vi "niRFUtil LCAPI Copy 1D Array (1 I8).vi"(0 "Source0 1D Array (I8)":i8[](array[numeric]), 11 "error in (no error)":errorcluster, 12 "Data Copy Descriptor":u64) -> (4 "Source0 1D Array (I8) Out":i8[](array[numeric]), 15 "error out":errorcluster)   [LabVIEW 2015, in "niRFUtil.lvlib"]
uses:
  niRFUtil.lvlib
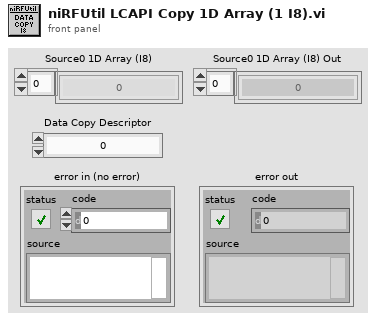
[diagram p1: front panel]
types:
  T1 = cluster{"status":bool, "return type":i32, "errorString":string}
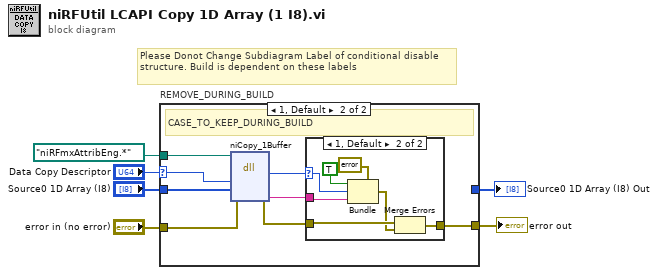
[diagram p0: block diagram]
diagram:
  # "Please Donot Change Subdiagram Label of conditional disable structure. Build is dependent on these labels"
  n1 = case "REMOVE_DURING_BUILD" shown="1, Default" "Data Copy Descriptor" {
    selector: "Data Copy Descriptor" -> [_ w10]
    tunnel: "error in (no error)" -> [w7 w16]
    tunnel: "Source0 1D Array (I8)" -> [w8 w15]
    tunnel: [w8 _] -> w3
    tunnel: [w7 w14] -> w2
    tunnel: path "niRFmxAttribEng.*" ("path in") -> [_ w9]
    frame 0 {
      # "Development"
    }
    frame 1, Default {
      # "CASE_TO_KEEP_DURING_BUILD"
      n2 = dll-call lib="niRFmxAttribEng.*" fn="niCopy_1Buffer"(path in=w9, error in=w16, "dataCopyDescriptor"=w10, "source"=w15) -> (error out=w11:errorcluster, "return type"=w12:i32, "errorString"=w13:string)  [unwired: 4 in, 1 out]
      n3 = case shown="1, Default" w12 {
        selector: w12 -> [_ w23]
        tunnel: w13 -> [_ w22]
        tunnel: w11 -> [w17 w20]
        tunnel: [w17 w21] -> w14
        frame 0 {
        }
        frame 1, Default {
          n4 = Bundle(cluster=T1 {"status"=FALSE, "return type"=0, "errorString"=""}, "status"=TRUE, "return type"=w23, "errorString"=w22) -> (w19:T1)
          n5 = Merge Errors(w20, w19) -> (w21:errorcluster)
        }
      }
    }
  }
  "Source0 1D Array (I8) Out" <- w3
  "error out" <- w2
